vi "initialize.vi"(0 "HGF_Timing":refnum<class "HGF_Timing.lvclass">, 3 "initializationData":variant, 5 "error in (no error)":errorcluster, 7 "binaryString":string, 8 "I8 Array":i8[](array[numeric]), 9 "prependSize? (T)":bool, 11 "byteOrder (0:big-endian, network order)":T1(ring)) -> (14 "dup HGF_Timing":refnum<class "HGF_Timing.lvclass">, 17 "found?":bool, 19 "error out":errorcluster)   [LabVIEW 2014, in "HGF_BaseClasses.lvlib" / "HGF_Timing.lvclass"]
doc: "This is a dynamic dispatch VI to be implemented by child classes to initialize their attributes.\n\n<B>Recommendation:</B> Use Variant for initialization data."
uses:
  HGF_Timing.lvclass
  HGF_Event/HGF_Event.lvclass
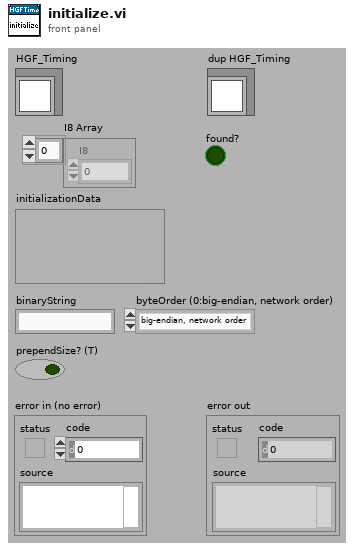
[diagram p1: front panel]
types:
  T1 = enum16{"big-endian, network order", "native, host order", "little-endian"}
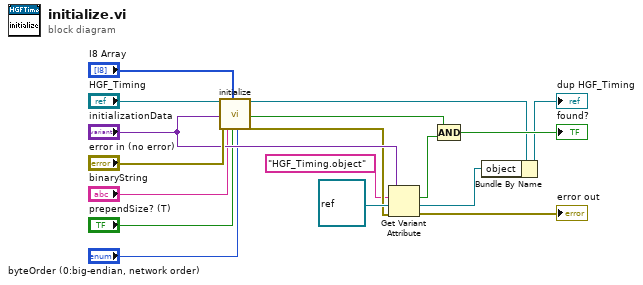
[diagram p0: block diagram]
diagram:
  n1 = call-parent "initialize.vi"("HGF_Event"="HGF_Timing", "initializationData"="initializationData", "error in (no error)"="error in (no error)", "binaryString"="binaryString", "I8 Array"="I8 Array", "prependSize? (T)"="prependSize? (T)", "byteOrder (0:big-endian, network order)"="byteOrder (0:big-endian, network order)") -> ("dup HGF_Event"=w6:refnum<class "HGF_Timing.lvclass">, "found?"=w9:bool, "error out"=w12:errorcluster)  [unwired: 1 in, 9 out]
  n2 = Get Variant Attribute(Variant="initializationData", name="HGF_Timing.object", default value (empty Variant)=refnum<class> refnum ("LabVIEW Object"), error in=w12) -> (found=w10:bool, value=w4:refnum<class>, error out=→"error out":errorcluster)  [unwired: 1 out]
  n3 = Compound Arithmetic op=AND(w9, w10) -> (→"found?":bool)
  n4 = Bundle By Name(cluster=w6, "object"=w4) -> (→"dup HGF_Timing":refnum<class "HGF_Timing.lvclass">)
